vi "Read gRPC Device Interface.vi"(8 "error in (no error)":errorcluster, 11 "instrument in":refnum<class "Instrument.lvclass">) -> (0 "error out":errorcluster, 2 "grpc device interface":string, 3 "instrument out":refnum<class "Instrument.lvclass">)   [LabVIEW 2020, in "MeasurementLink Instrument.lvlib" / "Instrument.lvclass"]
doc: "Returns the grpc-device interface that will be used to query the MeasurmentLink DiscoveryService for the address and port of the grpc-device server."
uses:
  Instrument.lvclass
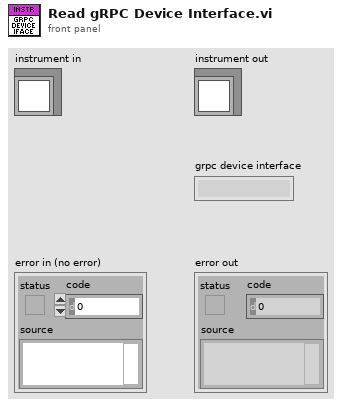
[diagram p1: front panel]
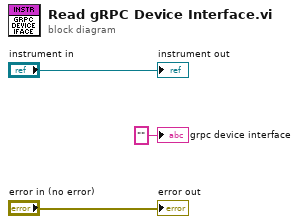
[diagram p0: block diagram]
diagram:
  "error out" <- "error in (no error)"
  "instrument out" <- "instrument in"
  "grpc device interface" <- "" ("grpc device interface")
